vi "Acquisition Hold Off State_Actions.vi"(9 "Pre-Trigger Samples":u16, 11 "Hold-Off Time Done?":bool=TRUE) -> (3 "State Output":T1)   [LabVIEW 2012]
uses:
  State Execution Output.ctl
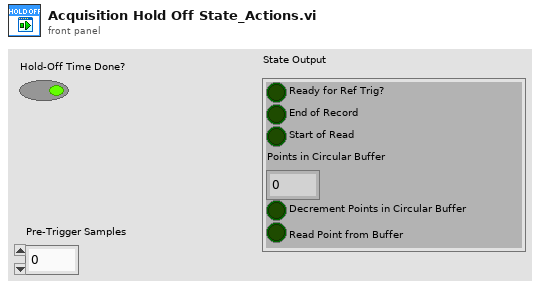
[diagram p1: front panel]
types:
  T1 = typedef "State Execution Output.ctl" = cluster{"Ready for Ref Trig?":bool, "End of Record":bool, "Start of Read":bool, "Points in Circular Buffer":u16, "Decrement Points in Circular Buffer":bool, "Read Point from Buffer":bool}
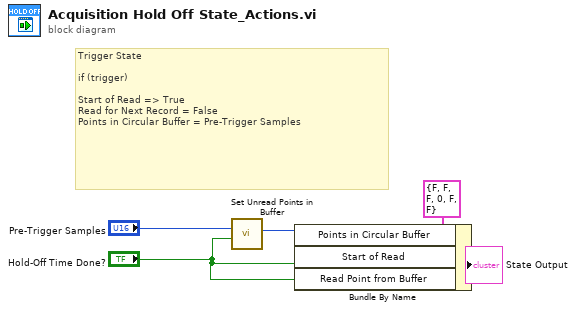
[diagram p0: block diagram]
diagram:
  # "Trigger State\n\nif (trigger)\n\nStart of Read => True\nRead for Next Record = False\nPoints in Circular Buffer = Pre-Trigger Samples"
  n1 = call "Set Unread Points in Buffer.vi"("Set"="Hold-Off Time Done?", "Value"="Pre-Trigger Samples") -> ("Value"=w3:u16)  [unwired: 9 in]
  n2 = Bundle By Name(cluster=T1 {"Ready for Ref Trig?"=FALSE, "End of Record"=FALSE, "Start of Read"=FALSE, "Points in Circular Buffer"=0, "Decrement Points in Circular Buffer"=FALSE, "Read Point from Buffer"=FALSE} ("State Execution Outputs"), "Points in Circular Buffer"=w3, "Start of Read"="Hold-Off Time Done?", "Read Point from Buffer"="Hold-Off Time Done?") -> (→"State Output":T1)
